vi "_Found Node with Key Value.vi"(4 "error in (no error)":errorcluster, 5 "Value":string, 6 "Key":string, 7 "nodes":refnum<k20>[](array[refnum])) -> (0 "error out":errorcluster, 2 "Found":bool, 3 "node out":refnum<k20>)   [LabVIEW 2012]
uses:
  <vilib>/xml/Close Reference(Node).vi
  <vilib>/xml/NI_XML.lvlib
  <resource>/objmgr/DOMUserDefRef.rc
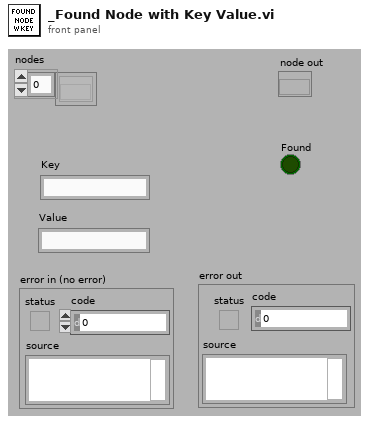
[diagram p1: front panel]
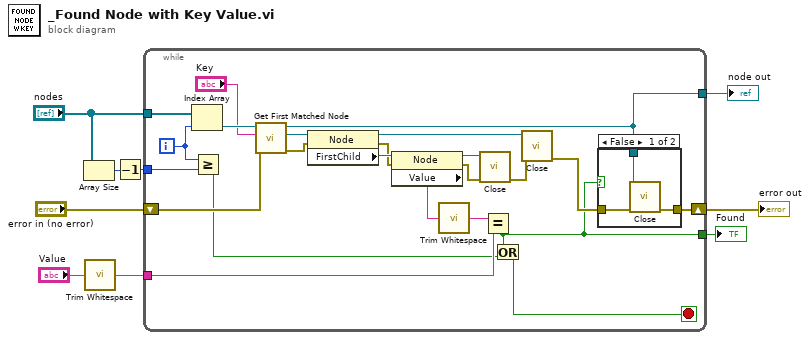
[diagram p0: block diagram]
diagram:
  n1 = Array Size(array="nodes") -> (size(s)=w8:i32)
  n2 = call <vilib>:"Trim Whitespace.vi"("string"="Value") -> ("trimmed string"=w5:string)  [unwired: 1 in]
  n3 = Decrement(x=w8) -> (x-1=w1:i32)
  n4 = while {
    tunnel: "nodes" -> [w32]
    tunnel: w1 -> [w30]
    shift-right: [w11] -> w2
    shift-left: "error in (no error)" -> [w27]
    tunnel: w5 -> [w18]
    tunnel: [w10] -> w3
    tunnel: [w12] -> w4
    i -> [w31]
    stop <- w14 stop-if-true
    n5 = Index Array(array=w32, index=w31) -> (element=w29:refnum<k20>)
    n6 = Greater Or Equal?(x=w31, y=w30) -> (x >= y?=w15:bool)
    n7 = call <vilib>:"Get First Matched Node.vi"("error in (no error)"=w27, "XPath expression"="Key", "node in"=w29) -> ("error out"=w24:errorcluster, "node result"=w26:refnum<k20>, "node out"=w12:refnum<k20>)  [unwired: 6 in]
    n8 = property class="Node"(reference=w26, error in=w24) -> (reference out=w17:refnum<k20>, error out=w23:errorcluster, "FirstChild"=w25:refnum<k20>)
    n9 = property class="Node"(reference=w25, error in=w23) -> (reference out=w22:refnum<k20>, error out=w21:errorcluster, "Value"=w20:string)
    n10 = call <vilib>:"Trim Whitespace.vi"("string"=w20) -> ("trimmed string"=w19:string)  [unwired: 1 in]
    n11 = call-poly <vilib>:"Close.vi"("error in (no error)"=w21, "node"=w22) -> ("error out"=w16:errorcluster)  [unwired: 7 in]
    n12 = Equal?(x=w19, y=w18) -> (x = y?=w10:bool)
    n13 = Or(x=w10, y=w15) -> (x .or. y?=w14:bool)
    n14 = call-poly <vilib>:"Close.vi"("error in (no error)"=w16, "node"=w17) -> ("error out"=w13:errorcluster)  [unwired: 7 in]
    n15 = case shown="False" w10 {
      tunnel: w13 -> [w35 w36]
      tunnel: w12 -> [w34 _]
      tunnel: [w33 w36] -> w11
      frame False {
        n16 = call-poly <vilib>:"Close.vi"("error in (no error)"=w35, "node"=w34) -> ("error out"=w33:errorcluster)  [unwired: 7 in]
      }
      frame True {
      }
    }
  }
  "node out" <- w4
  "error out" <- w2
  "Found" <- w3
